vi "Write Comments.vi"(8 "error in (no error)":errorcluster, 10 "Comments":string, 11 "LVtoITX in":refnum<class "LV to ITX.lvclass">) -> (0 "error out":errorcluster, 3 "LVtoITX out":refnum<class "LV to ITX.lvclass">)   [LabVIEW 2016, in "LV to ITX.lvclass"]
uses:
  LV to ITX.lvclass
  LV to ITX.lvclass/LV to ITX.ctl
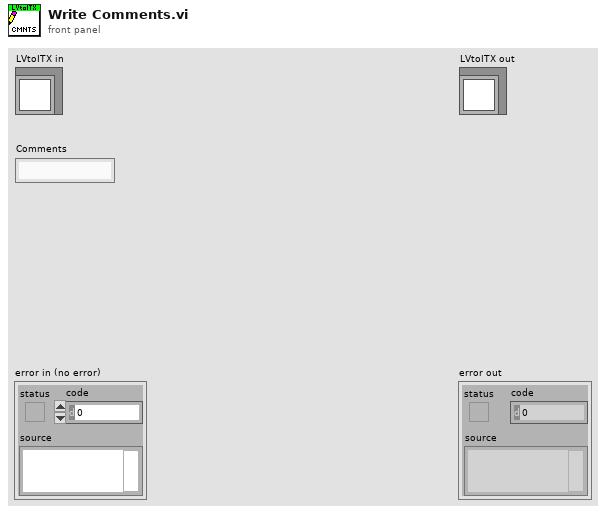
[diagram p1: front panel]
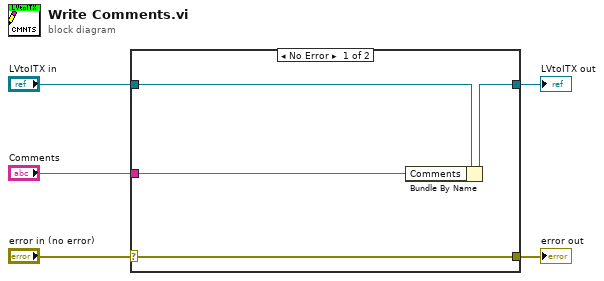
[diagram p0: block diagram]
diagram:
  n1 = case shown="No Error" "error in (no error)" {
    selector: "error in (no error)" -> [w9 w10]
    tunnel: [w9 w10] -> w4
    tunnel: [w6 w11] -> w2
    tunnel: "LVtoITX in" -> [w8 w11]
    tunnel: "Comments" -> [w7 _]
    frame No Error {
      n2 = Bundle By Name(cluster=w8, "Comments"=w7) -> (w6:refnum<class "LV to ITX.lvclass">)
    }
    frame Error {
    }
  }
  "error out" <- w4
  "LVtoITX out" <- w2
